vi "STOP.vi"(8 "error in (no error)":errorcluster caption="entrée d'erreur (pas d'erreur)", 11 "VIS-IR en entrée":refnum<class "VIS-NIR.lvclass">) -> (0 "error out":errorcluster caption="sortie d'erreur", 3 "VIS-IR en sortie":refnum<class "VIS-NIR.lvclass">)   [LabVIEW 2015, in "VIS-NIR.lvclass"]
uses:
  VIS-NIR.lvclass
  GeneralFunctionality/GeneralFunctionality.lvclass/GeneralFunctionality.ctl
  GeneralFunctionality/GeneralFunctionality.lvclass
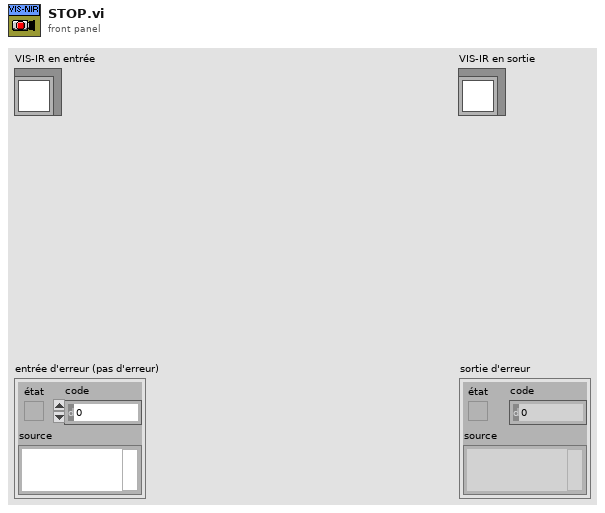
[diagram p1: front panel]
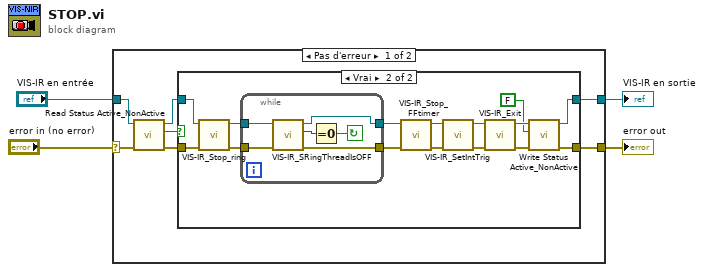
[diagram p0: block diagram]
diagram:
  n1 = case shown="Pas d'erreur" "error in (no error)" {
    selector: "error in (no error)" -> [w9 w36]
    tunnel: [w10 w36] -> w3
    tunnel: "VIS-IR en entrée" -> [w8 w35]
    tunnel: [w11 w35] -> w1
    frame No Error {
      n2 = call "Read Status Active_NonActive.vi"("error in (no error)"=w9, "GeneralFunctionality in"=w8) -> ("error out"=w5:errorcluster, "Status Active/NonActive"=w7:bool, "GeneralFunctionality out"=w6:refnum<class "VIS-NIR.lvclass">)  [unwired: 7 in]
      n3 = case shown="Vrai" w7 {
        tunnel: [w13 w18] -> w11
        tunnel: [w12 w19] -> w10
        tunnel: w6 -> [w13 w15]
        tunnel: w5 -> [w12 w14]
        frame False {
        }
        frame True {
          n4 = call "VIS-IR_Stop_ring.vi"("error in (no error)"=w14, "VIS-IR in"=w15) -> ("error out"=w27:errorcluster, "VIS-IR out"=w28:refnum<class "VIS-NIR.lvclass">)  [unwired: 8 in]
          n5 = while {
            tunnel: w28 -> [w32]
            tunnel: w27 -> [w33]
            tunnel: [w30] -> w26
            tunnel: [w29] -> w25
            stop <- w34 continue-if-true
            n6 = call "VIS-IR_SRingThreadIsOFF.vi"("error in (no error)"=w33, "VIS-IR in"=w32) -> ("error out"=w30:errorcluster, "ThreadIsOFF"=w31:u8, "VIS-IR out"=w29:refnum<class "VIS-NIR.lvclass">)  [unwired: 7 in]
            n7 = Equal To 0?(x=w31) -> (x = 0?=w34:bool)
          }
          n8 = call "VIS-IR_Stop_FFtimer.vi"("error in (no error)"=w26, "VIS-IR in"=w25) -> ("error out"=w23:errorcluster, "VIS-IR out"=w24:refnum<class "VIS-NIR.lvclass">)  [unwired: 8 in]
          n9 = call "VIS-IR_SetIntTrig.vi"("error in (no error)"=w23, "VIS-IR in"=w24) -> ("error out"=w21:errorcluster, "VIS-IR out"=w22:refnum<class "VIS-NIR.lvclass">)  [unwired: 8 in]
          n10 = call "VIS-IR_Exit.vi"("error in (no error)"=w21, "VIS-IR in"=w22) -> ("error out"=w20:errorcluster, "VIS-IR out"=w17:refnum<class "VIS-NIR.lvclass">)  [unwired: 8 in]
          n11 = call "Write Status Active_NonActive.vi"("error in (no error)"=w20, "Status Active/NonActive"=FALSE, "GeneralFunctionality in"=w17) -> ("error out"=w19:errorcluster, "GeneralFunctionality out"=w18:refnum<class "VIS-NIR.lvclass">)  [unwired: 7 in]
        }
      }
    }
    frame Error {
    }
  }
  "error out" <- w3
  "VIS-IR en sortie" <- w1
